vi "Authorization Write oasis License File.vi"(8 "error in (no error)":errorcluster, 9 "Authorization":T1, 11 "Path":path) -> (0 "error out":errorcluster)   [LabVIEW 2011]
uses:
  Authorization XML.ctl
panel:
  in  "String":string
  out "appended path":path
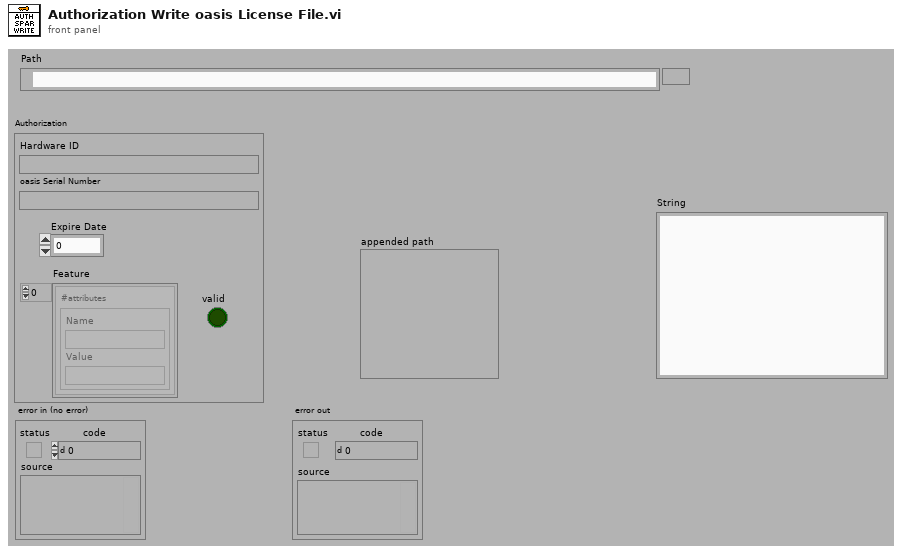
[diagram p1: front panel]
types:
  T1 = typedef "Authorization XML.ctl" = cluster{"Hardware ID":string, "oasis Serial Number":string, "Feature":cluster{"#attributes":cluster{"Name":string, "Value":string}}[], "valid":bool, "Expire Date":dbl}
  T2 = enum16{"open", "replace", "create", "open or create", "replace or create", "replace or create with confirmation"}
  T3 = cluster{"#attributes":cluster{"Name":string, "Value":string}}[]
  T4 = cluster{"#attributes":cluster{"Name":string, "Value":string}}
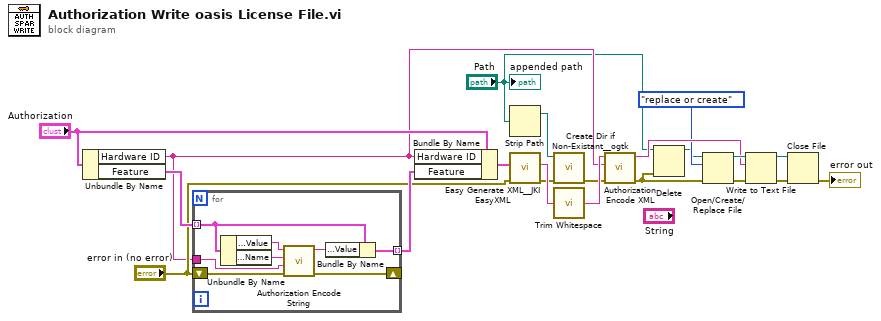
[diagram p0: block diagram]
diagram:
  n1 = Unbundle By Name("Authorization") -> ("Hardware ID"=w5:string, "Feature"=w10:T3)
  n2 = for {
    tunnel: w10 -> [w29] mode=indexing
    tunnel: [w28] -> w9 mode=indexing
    shift-right: [w26] -> _
    shift-left: "error in (no error)" -> [w27]
    tunnel: w5 -> [w22]
    n3 = Unbundle By Name(w29) -> ("#attributes.Value"=w24:string, "#attributes.Name"=w25:string)
    n4 = call "Authorization Encode String.vi"("error in (no error)"=w27, "Volume Serial Number"=w22, "Property Name"=w25, "Decoded String"=w24) -> ("error out"=w26:errorcluster, "Encoded String"=w23:string)  [unwired: 6 in]
    n5 = Bundle By Name(cluster=w29, "#attributes.Value"=w23) -> (w28:T4)
  }
  n6 = Bundle By Name(cluster="Authorization", "Hardware ID"=w5, "Feature"=w9) -> (w14:T1)
  n7 = Strip Path(path="Path") -> (stripped path=w4:path)  [unwired: 1 out]
  n8 = call <vilib>:"Easy Generate XML__JKI EasyXML.vi"("error in (no error)"="error in (no error)", "LabVIEW Data"=w14) -> ("error out"=w3:errorcluster, "XML String"=w13:string)  [unwired: 8 in]
  n9 = call <userlib>:"Create Dir if Non-Existant__ogtk.vi"("error in (no error)"=w3, "Directory Path"=w4) -> ("error out"=w2:errorcluster)  [unwired: 7 in, 2 out]
  n10 = call <vilib>:"Trim Whitespace.vi"("string"=w13) -> ("trimmed string"=w12:string)  [unwired: 1 in]
  n11 = call "Authorization Encode XML.vi"("error in (no error)"=w2, "Volume Serial Number"=w5, "Decoded XML String"=w12) -> ("error out"=w7:errorcluster, "Encoded XML String"=w16:string)  [unwired: 7 in]
  n12 = Delete(path (use dialog)="Path", error in=w7) -> (deleted path=w6:path)  [unwired: 3 in, 2 out]
  n13 = Open/Create/Replace File(file path (use dialog)=w6, error in=w7, operation (0:open)=T2."replace or create") -> (refnum out=w17:refnum<file>, error out=w21:errorcluster)  [unwired: 3 in, 1 out]
  n14 = Write to Text File(file (use dialog)=w17, text=w16, error in=w21) -> (refnum out=w18:refnum<file>, error out=w20:errorcluster)  [unwired: 1 in, 1 out]
  n15 = Close File(refnum=w18, error in=w20) -> (error out=→"error out":errorcluster)  [unwired: 1 out]
  "appended path" <- "Path"
